vi "固定站流程平行样自动启动.vi"(11 "参数":T1) -> ()   [LabVIEW 2016, in "质控单元.lvlib"]
panel:
  out "枚举":enum16{"初始化", "采配水启动", "等待", "配水", "排水", "结束"}(ring)
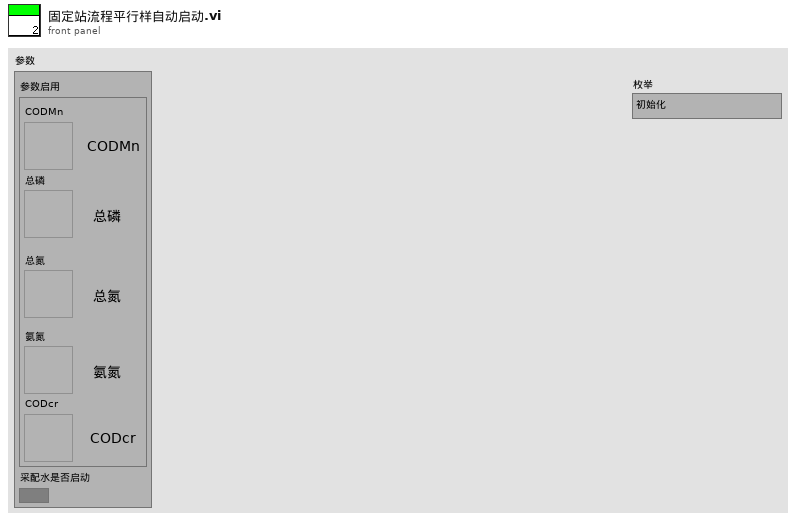
[diagram p1: front panel]
types:
  T1 = cluster{"参数启用":cluster{"CODMn":bool, "总磷":bool, "总氮":bool, "氨氮":bool, "CODcr":bool}, "采配水是否启动":bool}
  T2 = cluster{"命令":string, cluster{"starting address":u16, "holding register value":u16}}
  T3 = typedef "质控单元.lvlib/平行样测试流程.ctl" = enum16{"待机", "第一次水样测试启动", "第一次水样测试中", "第二次水样测试启动", "第二次水样测试中", "存储平行样测试数据", "结束"}
  T4 = cluster{"站号":u16, "量程切换":enum32{"H", "L", "AUTO"}, "控制命令":enum16{"启动测量", "标样核查", "零点核查", "跨度核查", "空白测试", "平行样测试", "加标回收", "空白校准", "标样校准", "初始化（清洗）", "停止测试", "仪器重启", "校时", "模式设置", "测量间隔设置"}, "模式设置":enum16{"待机", "连续模式", "周期模式", "定点模式", "受控模式", "手动模式"}, "测量间隔":u16}
  T5 = cluster{"时间标识":timestamp, "设备":string, "日志信息":string}
  T6 = enum16{"空闲", "水样测试", "标样核查", "零点核查", "跨度核查", "空白测试", "平行样测试", "加标回收", "空白校准", "标样校准", "初始化（清洗）"}
  T7 = cluster{"测量模式":enum16{"水样测量", "标样核查", "零点核查", "跨度核查", "空白测试", "加标回收", "平行样", "校零", "校标"}}
  T8 = cluster{"时间标识":timestamp, "设备":string, "日志信息":string, "流程参数":string}
  T9 = cluster{"R0":i16, "R1":i16, "R2":i16, "R3":i16, "R4":i16, "R5":i16, "R6":i16, "R7":i16, "R8":i16, "R9":i16, "R10":i16, "R11":i16, "R12":i16, "R13":i16, "R14":i16, "R15":i16, "R16":i16, "R17":i16, "R18":i16, "R19":i16, "R20":i16, "R21":i16, "R22":i16, "R23":i16, "R24":i16, "R25":i16, "R26":i16, "R27":i16, "R28":i16, "R29":i16, "R30":i16, "R31":i16, "R32":i16, "R33":i16, "R34":i16, "R35":i16, "R36":i16, "R37":i16, "R38":i16, "R39":i16, "R40":i16, "R41":i16, "R42":i16, "R43":i16, "R44":i16, "R45":i16, "R46":i16, "R47":i16, "R48":i16, "R49":i16, "R50":i16, "R51":i16, "R52":i16, "R53":i16, "R54":i16, "R55":i16, "R56":i16}
  T10 = cluster{"时间标识":timestamp, "参数":string, "数据类型":string, "第一次水样浓度值":sgl, "第二次水样测试时间":timestamp, "第二次水样浓度值":sgl}
  T11 = cluster{"系统时间":timestamp, "工作状态":enum16{"空闲", "水样测试", "标样核查", "零点核查", "跨度核查", "空白测试", "平行样测试", "加标回收", "空白校准", "标样校准", "初始化（清洗）"}, "测量模式":enum16{"待机", "连续模式", "周期模式", "定点模式", "受控模式", "手动模式"}, "告警代码":enum16{"无告警", "缺试剂告警", "缺水样告警", "缺蒸馏水告警", "缺标液告警", "仪表漏液告警", "标定异常告警", "超量程告警", "加热异常", "低试剂预警", "超上限告警", "超下限告警", "仪表内部其他异常", "滴定异常告警", "电极异常告警", "量程切换告警", "参数设置告警", "PH电极电位异常", "电导率电极异常", "浊度光度异常", "溶解氧电极异常", "溶解氧光强异常", "温度异常告警", "PH异常告警", "溶解氧异常告警", "电导率异常告警", "浊度异常告警", "叶绿素异常告警", "藻密度异常告警", "蓝绿藻异常告警", "ORP异常告警", "氨氮异常告警", "清洁刷异常告警", "SD卡异常告警", "蓝牙异常告警", "Wifi异常告警", "流程异常告警"}, "故障代码":enum16{"无故障", "电机故障", "温度故障", "通讯故障", "滴定故障"}, "日志代码":u16, "软件版本":u16, "F0":sgl, "F1":sgl, "F2":sgl, "F3":sgl, "T":sgl, "H":sgl, "id":u16, "flowid":u16, "量程":u16, "总磷控温温度1":sgl, "营养盐控温温度2":sgl, "ADC":sgl}
  T12 = cluster{"因子编码":u32, "单位":u16, "标样参考值":sgl, "水样数据时间":timestamp, "水样实测值":sgl, "水样数据标识":string, "标样数据时间":timestamp, "标样实测值":sgl, "标样数据标识":string, "空白数据时间":timestamp, "空白实测值":sgl, "空白数据标识":string, "零点核查数据时间":timestamp, "零点核查实测值":sgl, "零点核查数据标识":string, "跨度核查数据时间":timestamp, "跨度核查实测值":sgl, "跨度核查数据标识":string, "加标回收数据时间":timestamp, "加标回收实测值":sgl, "加标回收数据标识":string, "平行样数据时间":timestamp, "平行样实测值":sgl, "平行样数据标识":string}
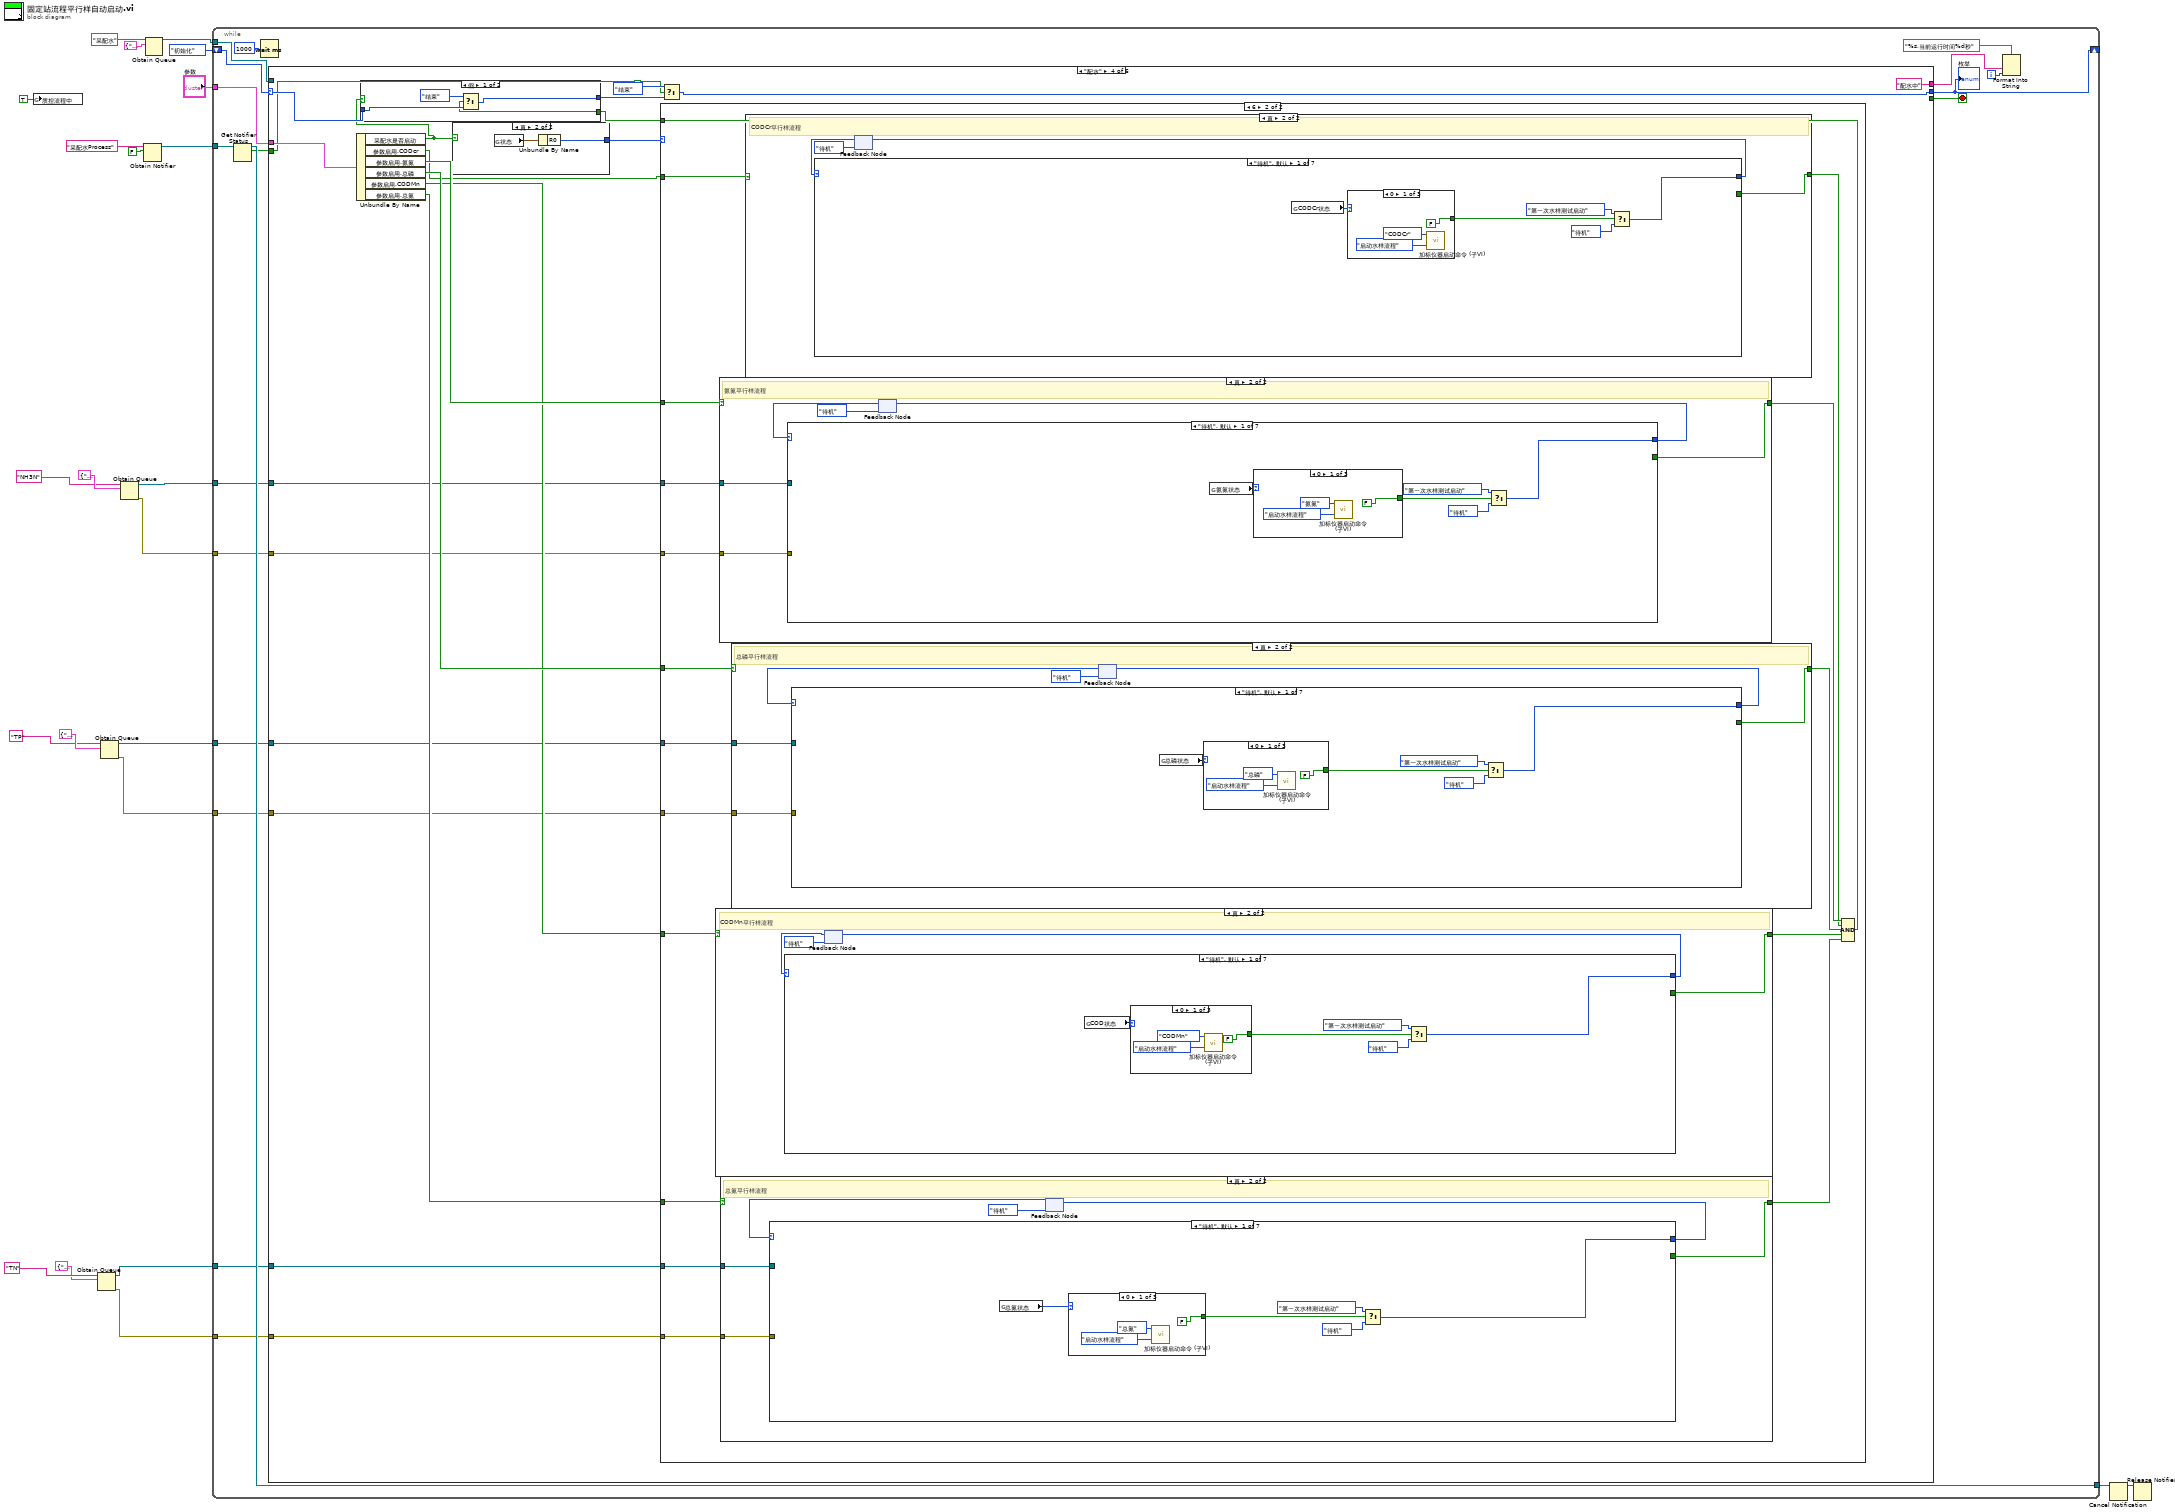
[diagram p0: block diagram]
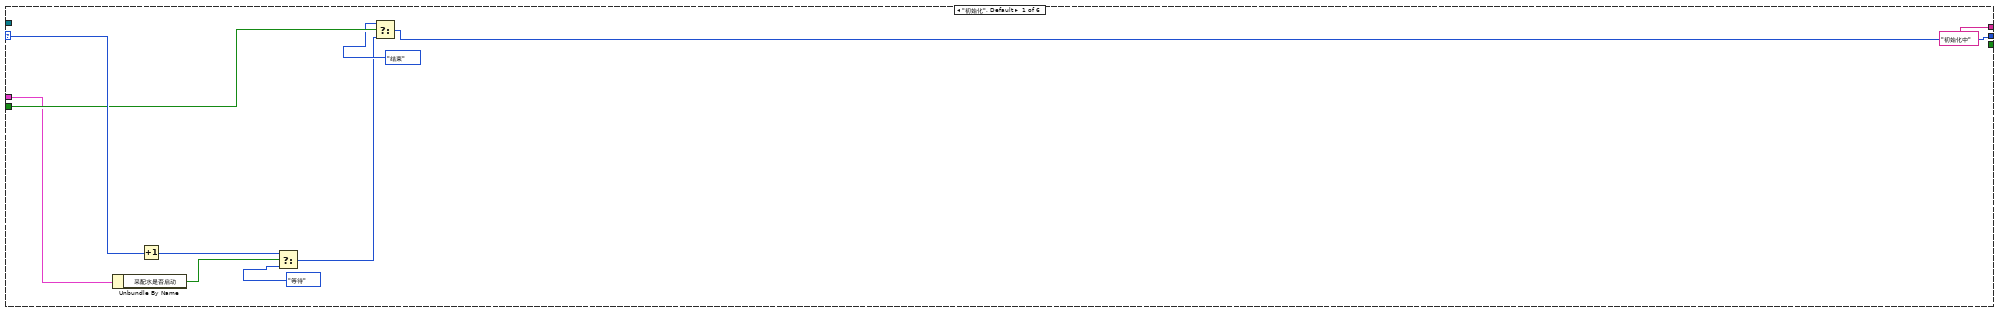
[diagram p2: hidden frame]
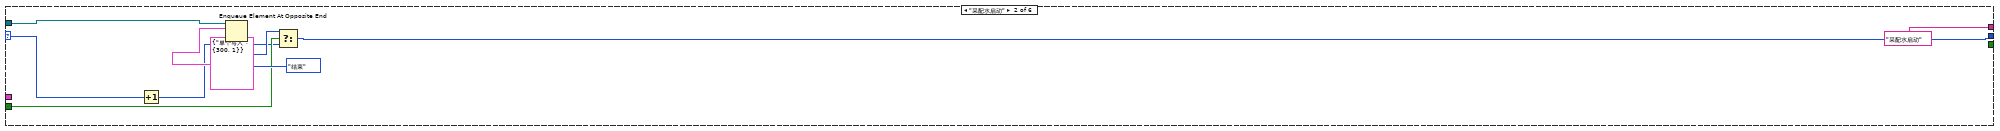
[diagram p3: hidden frame]
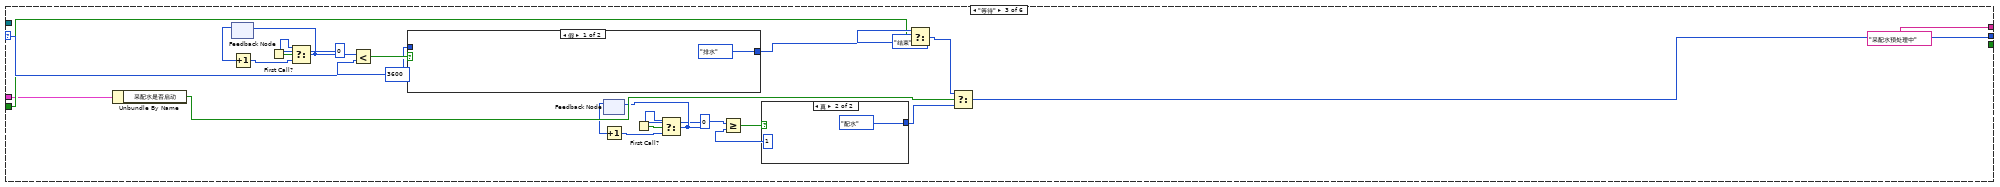
[diagram p4: hidden frame]
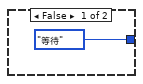
[diagram p5: hidden frame]
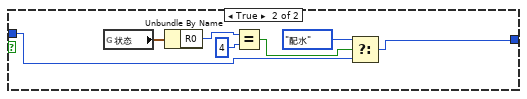
[diagram p6: hidden frame]
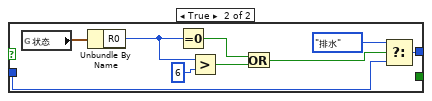
[diagram p7: hidden frame]
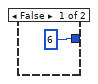
[diagram p8: hidden frame]
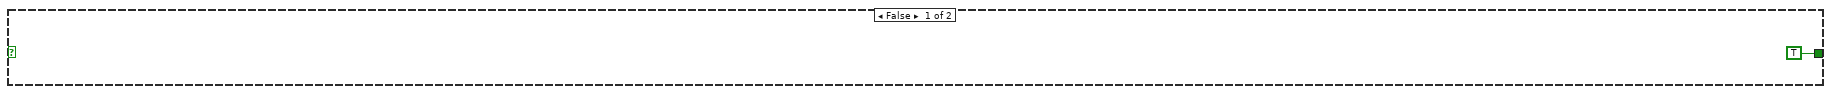
[diagram p10: hidden frame]
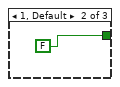
[diagram p11: hidden frame]
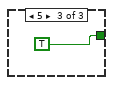
[diagram p12: hidden frame]
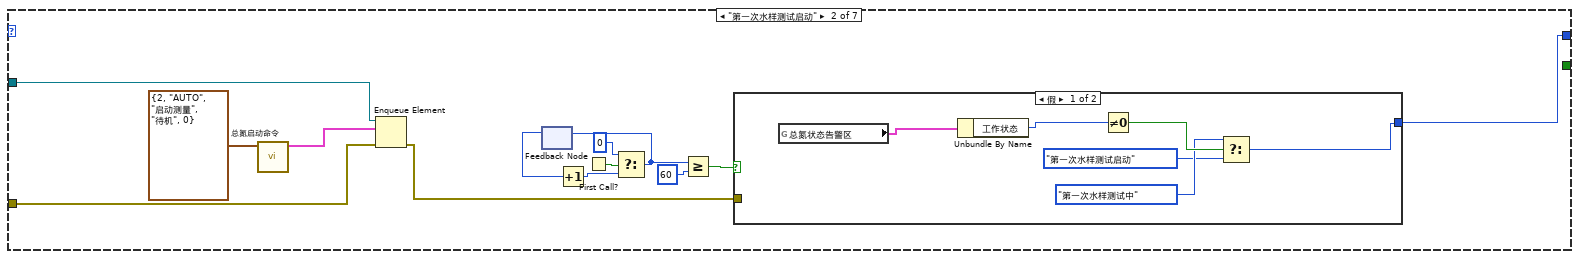
[diagram p13: hidden frame]
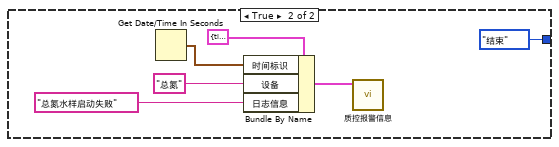
[diagram p14: hidden frame]
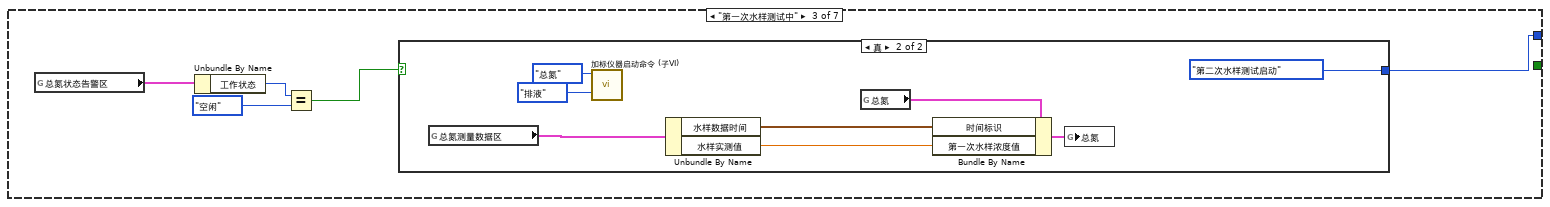
[diagram p15: hidden frame]
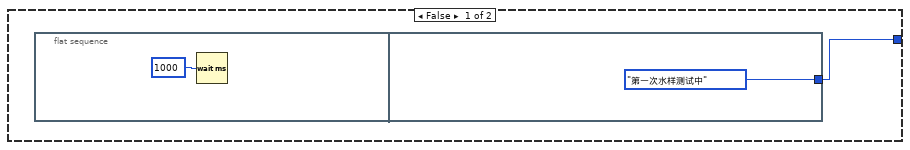
[diagram p16: hidden frame]
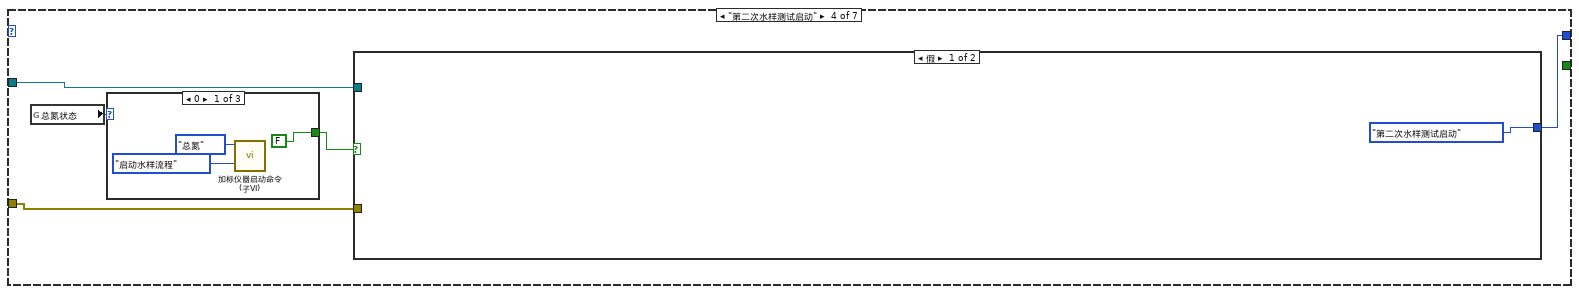
[diagram p17: hidden frame]
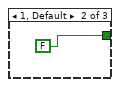
[diagram p18: hidden frame]
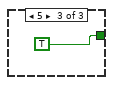
[diagram p19: hidden frame]
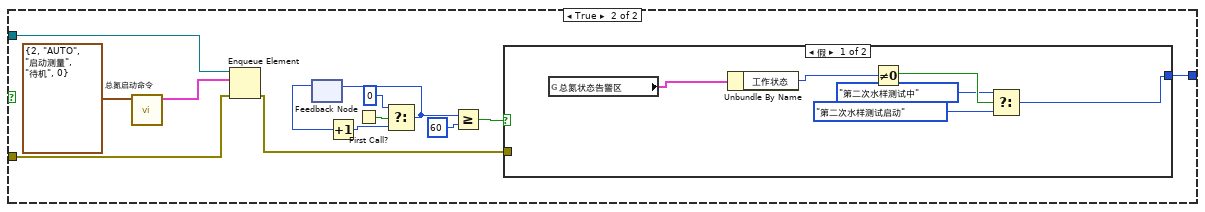
[diagram p20: hidden frame]
diagram:
  n1 = global write "质控测完标志全局 1.vi" "质控流程中"(TRUE ("质控流程中")) -> ()
  n2 = Obtain Queue(name (unnamed)="TN" ("名称（未命名）"), element data type=cluster{"命令":string, "data":variant} {"命令"="", "data"=variant}) -> (queue out=w3:refnum<queue>, error out=w2:errorcluster)  [unwired: 3 in, 1 out]
  n3 = Obtain Queue(name (unnamed)="TP" ("名称（未命名）"), element data type=cluster{"命令":string, "data":variant} {"命令"="", "data"=variant}) -> (queue out=w5:refnum<queue>, error out=w4:errorcluster)  [unwired: 3 in, 1 out]
  n4 = Obtain Queue(name (unnamed)="NH3N" ("名称（未命名）"), element data type=cluster{"命令":string, "data":variant} {"命令"="", "data"=variant}) -> (queue out=w7:refnum<queue>, error out=w6:errorcluster)  [unwired: 3 in, 1 out]
  n5 = Obtain Notifier(name (unnamed)="采配水Process" ("名称（未命名）"), notification data type=FALSE) -> (notifier out=w16:refnum<notifier>)  [unwired: 2 in, 2 out]
  n6 = Obtain Queue(name (unnamed)="采配水" ("名称（未命名）"), element data type=cluster{"命令":string, "数据":variant} {"命令"="", "数据"=variant}) -> (queue out=w21:refnum<queue>)  [unwired: 3 in, 2 out]
  n7 = while {
    tunnel: w21 -> [w41]
    shift-right: [w39] -> _
    shift-left: enum16{"初始化", "采配水启动", "等待", "配水", "排水", "结束"}."初始化" ("枚举") -> [w40]
    tunnel: "参数" -> [w37]
    tunnel: w16 -> [w36]
    tunnel: [w35] -> w15
    tunnel: w7 -> [w30]
    tunnel: w6 -> [w29]
    tunnel: w5 -> [w28]
    tunnel: w4 -> [w27]
    tunnel: w3 -> [w26]
    tunnel: w2 -> [w25]
    i -> [w32]
    stop <- w24 stop-if-true
    n8 = Get Notifier Status(notifier=w36) -> (notifier out=w35:refnum<notifier>, current notification=w31:bool)  [unwired: 1 in, 3 out]
    n9 = Wait (ms)(milliseconds to wait=u32 1000 ("等待时间（毫秒）")) -> ()  [unwired: 1 out]
    n10 = case shown="\"配水\"" w40 {
      selector: w40 -> [w51 w57 w81 w114 w707 w714]
      tunnel: w41 -> [_ w58 _ _ w708 _]
      tunnel: [w48 w52 w60 w111 w702 w713] -> w39
      tunnel: [_ _ _ _ _ TRUE] -> w24
      tunnel: w37 -> [w46 _ w71 w107 _ _]
      tunnel: ["初始化中" ("输入 1") "采配水启动" ("输入 1") "采配水预处理中" ("输入 1") "配水中" ("输入 1") "排水中" ("输入 1") "结束" ("输入 1")] -> w33
      tunnel: w31 -> [w49 w54 w73 w95 w704 _]
      tunnel: w30 -> [_ _ _ w102 _ _]
      tunnel: w29 -> [_ _ _ w101 _ _]
      tunnel: w28 -> [_ _ _ w100 _ _]
      tunnel: w27 -> [_ _ _ w99 _ _]
      tunnel: w26 -> [_ _ _ w98 _ _]
      tunnel: w25 -> [_ _ _ w97 _ _]
      frame "初始化", Default {
        n11 = Unbundle By Name(w46) -> ("采配水是否启动"=w45:bool)
        n12 = Increment(x=w51) -> (x+1=w44:enum16{"初始化", "采配水启动", "等待", "配水", "排水", "结束"})
        n13 = Select(t=w44, s=w45, f=enum16{"初始化", "采配水启动", "等待", "配水", "排水", "结束"}."等待") -> (s? t:f=w43:enum16{"初始化", "采配水启动", "等待", "配水", "排水", "结束"})
        n14 = Select(t=enum16{"初始化", "采配水启动", "等待", "配水", "排水", "结束"}."结束", s=w49, f=w43) -> (s? t:f=w48:enum16{"初始化", "采配水启动", "等待", "配水", "排水", "结束"})
      }
      frame "采配水启动" {
        n15 = Increment(x=w57) -> (x+1=w53:enum16{"初始化", "采配水启动", "等待", "配水", "排水", "结束"})
        n16 = Enqueue Element At Opposite End(queue=w58, element=T2 {"命令"="单个写入", {"starting address"=300, "holding register value"=1}} ("元素")) -> ()  [unwired: 2 in, 3 out]
        n17 = Select(t=enum16{"初始化", "采配水启动", "等待", "配水", "排水", "结束"}."结束", s=w54, f=w53) -> (s? t:f=w52:enum16{"初始化", "采配水启动", "等待", "配水", "排水", "结束"})
      }
      frame "等待" {
        n18 = Unbundle By Name(w71) -> ("采配水是否启动"=w70:bool)
        n19 = feedback #1() -> (w78:i32)  [unwired: 1 in]
        n20 = Increment(x=w78) -> (x+1=w77:i32)
        n21 = First Call?() -> (First Call?: T/F=w79:bool)
        n22 = Select(t=0, s=w79, f=w77) -> (s? t:f=w76:i32)
        n23 = feedback-in #1(w76) -> ()
        n24 = Less?(x=w76, y=3600) -> (x < y?=w82:bool)
        n25 = case shown="假" w82 {
          tunnel: w81 -> [_ w88]
          tunnel: [enum16{"初始化", "采配水启动", "等待", "配水", "排水", "结束"}."排水" ("枚举") w87] -> w72
          frame False {
          }
          frame True {
            n26 = global read "与采配水交互全局.vi" "状态"() -> (w93:T9)
            n27 = Unbundle By Name(w93) -> ("R0"=w92:i16)
            n28 = Equal?(x=w92, y=i16 4) -> (x = y?=w90:bool)
            n29 = Select(t=enum16{"初始化", "采配水启动", "等待", "配水", "排水", "结束"}."配水" ("枚举"), s=w90, f=w88) -> (s? t:f=w87:enum16{"初始化", "采配水启动", "等待", "配水", "排水", "结束"})
          }
        }
        n30 = feedback #2() -> (w66:i32)  [unwired: 1 in]
        n31 = Increment(x=w66) -> (x+1=w67:i32)
        n32 = First Call?() -> (First Call?: T/F=w65:bool)
        n33 = Select(t=0, s=w65, f=w67) -> (s? t:f=w68:i32)
        n34 = feedback-in #2(w68) -> ()
        n35 = Greater Or Equal?(x=w68, y=1) -> (x >= y?=w62:bool)
        n36 = case shown="真" w62 {
          tunnel: [enum16{"初始化", "采配水启动", "等待", "配水", "排水", "结束"}."等待" ("t") enum16{"初始化", "采配水启动", "等待", "配水", "排水", "结束"}."配水" ("t")] -> w61
          frame False {
          }
          frame True {
          }
        }
        n37 = Select(t=enum16{"初始化", "采配水启动", "等待", "配水", "排水", "结束"}."结束", s=w73, f=w72) -> (s? t:f=w69:enum16{"初始化", "采配水启动", "等待", "配水", "排水", "结束"})
        n38 = Select(t=w69, s=w70, f=w61) -> (s? t:f=w60:enum16{"初始化", "采配水启动", "等待", "配水", "排水", "结束"})
      }
      frame "配水" {
        n39 = Unbundle By Name(w107) -> ("采配水是否启动"=w96:bool, "参数启用.CODcr"=w106:bool, "参数启用.氨氮"=w110:bool, "参数启用.总磷"=w109:bool, "参数启用.CODMn"=w108:bool, "参数启用.总氮"=w105:bool)
        n40 = case shown="真" w96 {
          tunnel: [i16 6 ("R0") w129] -> w104
          frame False {
          }
          frame True {
            n41 = global read "与采配水交互全局.vi" "状态"() -> (w130:T9)
            n42 = Unbundle By Name(w130) -> ("R0"=w129:i16)
          }
        }
        n43 = case shown="6" w104 {
          tunnel: w110 -> [_ w147]
          tunnel: w109 -> [_ w146]
          tunnel: w108 -> [_ w143]
          tunnel: w106 -> [_ w142]
          tunnel: w105 -> [_ w139]
          tunnel: w102 -> [_ w137]
          tunnel: w101 -> [_ w136]
          tunnel: w100 -> [_ w135]
          tunnel: w99 -> [_ w134]
          tunnel: w98 -> [_ w133]
          tunnel: w97 -> [_ w132]
          tunnel: [_ w131] -> w94
          frame 0, Default {
          }
          frame 6 {
            n44 = case shown="真" w143 {
              tunnel: [TRUE w264] -> w140
              frame False {
              }
              frame True {
                # "CODMn平行样流程"
                n45 = feedback #3(平行样测试流程."待机") -> (w266:T3)
                n46 = case shown="\"待机\", 默认" w266 {
                  tunnel: [w267 w286 w300 w313 w343 平行样测试流程."结束" 平行样测试流程."结束"] -> w265
                  tunnel: [_ _ _ _ _ _ TRUE] -> w264
                  frame "待机", Default {
                    n47 = global read "加标回收状态全局变量.vi" "COD状态"() -> (w271:u16)
                    n48 = case shown="0" w271 {
                      tunnel: [FALSE ("s") FALSE ("s") TRUE ("s")] -> w270
                      frame 0 {
                        n49 = call "加标仪器启动命令 (子VI).vi"("启动命令"=enum16{"启动水样流程", "启动加标流程", "排液", "停止"}."启动水样流程", "仪器"=enum16{"", "氨氮", "总磷", "总氮", "CODMn", "CODCr"}."CODMn") -> ()  [unwired: 9 in, 1 out]
                      }
                      frame 1, Default {
                      }
                      frame 5 {
                      }
                    }
                    n50 = Select(t=平行样测试流程."第一次水样测试启动", s=w270, f=平行样测试流程."待机") -> (s? t:f=w267:T3)
                  }
                  frame "第一次水样测试启动" {
                    n51 = feedback #4() -> (w282:i32)  [unwired: 1 in]
                    n52 = Increment(x=w282) -> (x+1=w283:i32)
                    n53 = call "CODMn启动命令 (子VI).vi"("启动测量模式"=T7 {"测量模式"=enum."水样测量"}) -> ("错误输出"=w277:errorcluster)  [unwired: 10 in]
                    n54 = First Call?() -> (First Call?: T/F=w281:bool)
                    n55 = Select(t=0, s=w281, f=w283) -> (s? t:f=w284:i32)
                    n56 = feedback-in #4(w284) -> ()
                    n57 = Greater Or Equal?(x=w284, y=60) -> (x >= y?=w279:bool)
                    n58 = case shown="假" w279 {
                      tunnel: [w290 平行样测试流程."结束"] -> w286
                      tunnel: w277 -> [_ _]
                      frame False {
                        n59 = global read "与CODMn交互全局.vi" "多列列表框"() -> (w289:i32)
                        n60 = Not Equal To 0?(x=w289) -> (x != 0?=w291:bool)
                        n61 = Select(t=平行样测试流程."第一次水样测试中", s=w291, f=平行样测试流程."第一次水样测试启动") -> (s? t:f=w290:T3)
                      }
                      frame True {
                        n62 = Get Date/Time In Seconds() -> (seconds since 1Jan1904=w294:timestamp)
                        n63 = Bundle By Name(cluster=T5 {"时间标识"=timestamp(0 s since 1904-01-01), "设备"="", "日志信息"=""} ("data in"), "时间标识"=w294, "设备"="CODMn", "日志信息"="CODMn启动失败") -> (w292:T5)
                        n64 = call "质控报警信息.vi"("data in"=w292) -> ()  [unwired: 10 in, 1 out]
                      }
                    }
                  }
                  frame "第一次水样测试中" {
                    n65 = global read "与CODMn交互全局.vi" "多列列表框"() -> (w299:i32)
                    n66 = Equal To 0?(x=w299) -> (x = 0?=w298:bool)
                    n67 = case shown="真" w298 {
                      tunnel: [w301 平行样测试流程."第二次水样测试启动"] -> w300
                      frame False {
                        n68 = flat-sequence {
                          tunnel: [平行样测试流程."第一次水样测试中"] -> w301
                          frame #0 {
                            n69 = Wait (ms)(milliseconds to wait=u32 1000 ("等待时间（毫秒）")) -> ()  [unwired: 1 out]
                          }
                          frame #1 {
                          }
                        }
                      }
                      frame True {
                        n70 = global read "与CODMn交互全局.vi" "COD浓度（mg/L)"() -> (w306:dbl)
                        n71 = global read "与CODMn交互全局.vi" "水样启动时间"() -> (w307:timestamp)
                        n72 = global read "平行样测试全局变量.vi" "CODMn"() -> (w309:T10)
                        n73 = Bundle By Name(cluster=w309, "时间标识"=w307, "第一次水样浓度值"=w306) -> (w308:T10)
                        n74 = global write "平行样测试全局变量.vi" "CODMn"(w308) -> ()
                        n75 = call "加标仪器启动命令 (子VI).vi"("启动命令"=enum16{"启动水样流程", "启动加标流程", "排液", "停止"}."排液", "仪器"=enum16{"", "氨氮", "总磷", "总氮", "CODMn", "CODCr"}."CODMn") -> ()  [unwired: 9 in, 1 out]
                      }
                    }
                  }
                  frame "第二次水样测试启动" {
                    n76 = global read "加标回收状态全局变量.vi" "COD状态"() -> (w312:u16)
                    n77 = case shown="0" w312 {
                      tunnel: [FALSE ("s") FALSE ("s") TRUE ("s")] -> w311
                      frame 0 {
                        n78 = call "加标仪器启动命令 (子VI).vi"("启动命令"=enum16{"启动水样流程", "启动加标流程", "排液", "停止"}."启动水样流程", "仪器"=enum16{"", "氨氮", "总磷", "总氮", "CODMn", "CODCr"}."CODMn") -> ()  [unwired: 9 in, 1 out]
                      }
                      frame 1, Default {
                      }
                      frame 5 {
                      }
                    }
                    n79 = case shown="真" w311 {
                      tunnel: [平行样测试流程."第二次水样测试启动" w324] -> w313
                      frame False {
                      }
                      frame True {
                        n80 = feedback #5() -> (w320:i32)  [unwired: 1 in]
                        n81 = Increment(x=w320) -> (x+1=w321:i32)
                        n82 = First Call?() -> (First Call?: T/F=w319:bool)
                        n83 = call "CODMn启动命令 (子VI).vi"("启动测量模式"=T7 {"测量模式"=enum."水样测量"}) -> ("错误输出"=w315:errorcluster)  [unwired: 10 in]
                        n84 = Select(t=0, s=w319, f=w321) -> (s? t:f=w322:i32)
                        n85 = feedback-in #5(w322) -> ()
                        n86 = Greater Or Equal?(x=w322, y=60) -> (x >= y?=w317:bool)
                        n87 = case shown="真" w317 {
                          tunnel: [w328 平行样测试流程."结束"] -> w324
                          tunnel: w315 -> [_ _]
                          frame False {
                            n88 = global read "与CODMn交互全局.vi" "多列列表框"() -> (w327:i32)
                            n89 = Not Equal To 0?(x=w327) -> (x != 0?=w329:bool)
                            n90 = Select(t=平行样测试流程."第二次水样测试中", s=w329, f=平行样测试流程."第二次水样测试启动") -> (s? t:f=w328:T3)
                          }
                          frame True {
                            n91 = Get Date/Time In Seconds() -> (seconds since 1Jan1904=w332:timestamp)
                            n92 = Bundle By Name(cluster=T5 {"时间标识"=timestamp(0 s since 1904-01-01), "设备"="", "日志信息"=""} ("data in"), "时间标识"=w332, "设备"="CODMn", "日志信息"="CODMn启动失败") -> (w330:T5)
                            n93 = call "质控报警信息.vi"("data in"=w330) -> ()  [unwired: 10 in, 1 out]
                          }
                        }
                      }
                    }
                  }
                  frame "第二次水样测试中" {
                    n94 = global read "与CODMn交互全局.vi" "多列列表框"() -> (w342:i32)
                    n95 = Equal To 0?(x=w342) -> (x = 0?=w341:bool)
                    n96 = case shown="真" w341 {
                      tunnel: [w344 平行样测试流程."存储平行样测试数据"] -> w343
                      frame False {
                        n97 = flat-sequence {
                          tunnel: [平行样测试流程."第二次水样测试中"] -> w344
                          frame #0 {
                            n98 = Wait (ms)(milliseconds to wait=u32 1000 ("等待时间（毫秒）")) -> ()  [unwired: 1 out]
                          }
                          frame #1 {
                          }
                        }
                      }
                      frame True {
                        n99 = global read "与CODMn交互全局.vi" "COD浓度（mg/L)"() -> (w349:dbl)
                        n100 = global read "与CODMn交互全局.vi" "水样启动时间"() -> (w350:timestamp)
                        n101 = global read "平行样测试全局变量.vi" "CODMn"() -> (w352:T10)
                        n102 = Bundle By Name(cluster=w352, "时间标识"=w350, "第一次水样浓度值"=w349) -> (w351:T10)
                        n103 = global write "平行样测试全局变量.vi" "CODMn"(w351) -> ()
                        n104 = call "加标仪器启动命令 (子VI).vi"("启动命令"=enum16{"启动水样流程", "启动加标流程", "排液", "停止"}."排液", "仪器"=enum16{"", "氨氮", "总磷", "总氮", "CODMn", "CODCr"}."CODMn") -> ()  [unwired: 9 in, 1 out]
                      }
                    }
                  }
                  frame "存储平行样测试数据" {
                    n105 = global read "平行样测试全局变量.vi" "CODMn"() -> (w354:T10)
                    n106 = call "平行样测试数据写入.vi"("data"=w354) -> ()  [unwired: 10 in, 1 out]
                  }
                  frame "结束" {
                  }
                }
                n107 = feedback-in #3(w265) -> ()
              }
            }
            n108 = case shown="真" w147 {
              tunnel: [TRUE w592] -> w145
              tunnel: w137 -> [_ w591]
              tunnel: w136 -> [_ w590]
              frame False {
              }
              frame True {
                # "氨氮平行样流程"
                n109 = feedback #6(平行样测试流程."待机") -> (w594:T3)
                n110 = case shown="\"待机\", 默认" w594 {
                  tunnel: [w596 w606 w635 w651 w686 平行样测试流程."结束" 平行样测试流程."结束"] -> w593
                  tunnel: [_ _ _ _ _ _ TRUE] -> w592
                  tunnel: w591 -> [_ w616 _ w650 _ _ _]
                  tunnel: w590 -> [_ w615 _ w649 _ _ _]
                  frame "待机", Default {
                    n111 = global read "加标回收状态全局变量.vi" "氨氮状态"() -> (w600:u16)
                    n112 = case shown="0" w600 {
                      tunnel: [FALSE ("s") FALSE ("s") TRUE ("s")] -> w599
                      frame 0 {
                        n113 = call "加标仪器启动命令 (子VI).vi"("启动命令"=enum16{"启动水样流程", "启动加标流程", "排液", "停止"}."启动水样流程", "仪器"=enum16{"", "氨氮", "总磷", "总氮", "CODMn", "CODCr"}."氨氮") -> ()  [unwired: 9 in, 1 out]
                      }
                      frame 1, Default {
                      }
                      frame 5 {
                      }
                    }
                    n114 = Select(t=平行样测试流程."第一次水样测试启动", s=w599, f=平行样测试流程."待机") -> (s? t:f=w596:T3)
                  }
                  frame "第一次水样测试启动" {
                    n115 = call "氨氮启动命令.vi"("参数"=T4 {"站号"=3, "量程切换"=enum."AUTO", "控制命令"=enum."启动测量", "模式设置"=enum."受控模式", "测量间隔"=0}) -> ("启动命令"=w618:cluster{"命令":string, "data":variant})  [unwired: 10 in]
                    n116 = Enqueue Element(queue=w616, element=w618, error in (no error)=w615) -> (error out=w607:errorcluster)  [unwired: 1 in, 2 out]
                    n117 = feedback #7() -> (w611:i32)  [unwired: 1 in]
                    n118 = Increment(x=w611) -> (x+1=w612:i32)
                    n119 = First Call?() -> (First Call?: T/F=w610:bool)
                    n120 = Select(t=0, s=w610, f=w612) -> (s? t:f=w613:i32)
                    n121 = feedback-in #7(w613) -> ()
                    n122 = Greater Or Equal?(x=w613, y=60) -> (x >= y?=w608:bool)
                    n123 = case shown="假" w608 {
                      tunnel: [w623 平行样测试流程."结束"] -> w606
                      tunnel: w607 -> [_ _]
                      frame False {
                        n124 = global read "与氨氮交互全局.vi" "氨氮状态告警区"() -> (w619:T11)
                        n125 = Unbundle By Name(w619) -> ("工作状态"=w620:T6)
                        n126 = Not Equal To 0?(x=w620) -> (x != 0?=w624:bool)
                        n127 = Select(t=平行样测试流程."第一次水样测试中", s=w624, f=平行样测试流程."第一次水样测试启动") -> (s? t:f=w623:T3)
                      }
                      frame True {
                        n128 = Get Date/Time In Seconds() -> (seconds since 1Jan1904=w627:timestamp)
                        n129 = Bundle By Name(cluster=T5 {"时间标识"=timestamp(0 s since 1904-01-01), "设备"="", "日志信息"=""} ("data in"), "时间标识"=w627, "设备"="氨氮", "日志信息"="氨氮水样启动失败") -> (w625:T5)
                        n130 = call "质控报警信息.vi"("data in"=w625) -> ()  [unwired: 10 in, 1 out]
                      }
                    }
                  }
                  frame "第一次水样测试中" {
                    n131 = global read "与氨氮交互全局.vi" "氨氮状态告警区"() -> (w634:T11)
                    n132 = Unbundle By Name(w634) -> ("工作状态"=w632:T6)
                    n133 = Equal?(x=w632, y=T6."空闲" ("工作状态")) -> (x = y?=w631:bool)
                    n134 = case shown="真" w631 {
                      tunnel: [w636 平行样测试流程."第二次水样测试启动"] -> w635
                      frame False {
                        n135 = flat-sequence {
                          tunnel: [平行样测试流程."第一次水样测试中"] -> w636
                          frame #0 {
                            n136 = Wait (ms)(milliseconds to wait=u32 1000 ("等待时间（毫秒）")) -> ()  [unwired: 1 out]
                          }
                          frame #1 {
                          }
                        }
                      }
                      frame True {
                        n137 = call "加标仪器启动命令 (子VI).vi"("启动命令"=enum16{"启动水样流程", "启动加标流程", "排液", "停止"}."排液", "仪器"=enum16{"", "氨氮", "总磷", "总氮", "CODMn", "CODCr"}."氨氮") -> ()  [unwired: 9 in, 1 out]
                        n138 = global read "与氨氮交互全局.vi" "氨氮测量数据区"() -> (w643:T12)
                        n139 = Unbundle By Name(w643) -> ("水样数据时间"=w642:timestamp, "水样实测值"=w641:sgl)
                        n140 = global read "平行样测试全局变量.vi" "氨氮"() -> (w645:T10)
                        n141 = Bundle By Name(cluster=w645, "时间标识"=w642, "第一次水样浓度值"=w641) -> (w644:T10)
                        n142 = global write "平行样测试全局变量.vi" "氨氮"(w644) -> ()
                      }
                    }
                  }
                  frame "第二次水样测试启动" {
                    n143 = global read "加标回收状态全局变量.vi" "氨氮状态"() -> (w648:u16)
                    n144 = case shown="0" w648 {
                      tunnel: [FALSE ("s") FALSE ("s") TRUE ("s")] -> w647
                      frame 0 {
                        n145 = call "加标仪器启动命令 (子VI).vi"("启动命令"=enum16{"启动水样流程", "启动加标流程", "排液", "停止"}."启动水样流程", "仪器"=enum16{"", "氨氮", "总磷", "总氮", "CODMn", "CODCr"}."氨氮") -> ()  [unwired: 9 in, 1 out]
                      }
                      frame 1, Default {
                      }
                      frame 5 {
                      }
                    }
                    n146 = case shown="真" w647 {
                      tunnel: [平行样测试流程."第二次水样测试启动" w662] -> w651
                      tunnel: w650 -> [_ w659]
                      tunnel: w649 -> [_ w658]
                      frame False {
                      }
                      frame True {
                        n147 = call "氨氮启动命令.vi"("参数"=T4 {"站号"=3, "量程切换"=enum."AUTO", "控制命令"=enum."启动测量", "模式设置"=enum."受控模式", "测量间隔"=0}) -> ("启动命令"=w661:cluster{"命令":string, "data":variant})  [unwired: 10 in]
                        n148 = Enqueue Element(queue=w659, element=w661, error in (no error)=w658) -> ()  [unwired: 1 in, 3 out]
                        n149 = feedback #8() -> (w666:i32)  [unwired: 1 in]
                        n150 = Increment(x=w666) -> (x+1=w667:i32)
                        n151 = First Call?() -> (First Call?: T/F=w665:bool)
                        n152 = Select(t=0, s=w665, f=w667) -> (s? t:f=w668:i32)
                        n153 = feedback-in #8(w668) -> ()
                        n154 = Greater Or Equal?(x=w668, y=60) -> (x >= y?=w663:bool)
                        n155 = case shown="假" w663 {
                          tunnel: [w672 平行样测试流程."结束"] -> w662
                          frame False {
                            n156 = global read "与氨氮交互全局.vi" "氨氮状态告警区"() -> (w675:T11)
                            n157 = Unbundle By Name(w675) -> ("工作状态"=w671:T6)
                            n158 = Not Equal To 0?(x=w671) -> (x != 0?=w670:bool)
                            n159 = Select(t=平行样测试流程."第二次水样测试中", s=w670, f=平行样测试流程."第二次水样测试启动") -> (s? t:f=w672:T3)
                          }
                          frame True {
                            n160 = Get Date/Time In Seconds() -> (seconds since 1Jan1904=w678:timestamp)
                            n161 = Bundle By Name(cluster=T5 {"时间标识"=timestamp(0 s since 1904-01-01), "设备"="", "日志信息"=""} ("data in"), "时间标识"=w678, "设备"="氨氮", "日志信息"="氨氮水样启动失败") -> (w677:T5)
                            n162 = call "质控报警信息.vi"("data in"=w677) -> ()  [unwired: 10 in, 1 out]
                          }
                        }
                      }
                    }
                  }
                  frame "第二次水样测试中" {
                    n163 = global read "与氨氮交互全局.vi" "氨氮状态告警区"() -> (w685:T11)
                    n164 = Unbundle By Name(w685) -> ("工作状态"=w683:T6)
                    n165 = Equal?(x=w683, y=T6."空闲" ("工作状态")) -> (x = y?=w682:bool)
                    n166 = case shown="真" w682 {
                      tunnel: [w687 平行样测试流程."存储平行样测试数据"] -> w686
                      frame False {
                        n167 = flat-sequence {
                          tunnel: [平行样测试流程."第二次水样测试中"] -> w687
                          frame #0 {
                            n168 = Wait (ms)(milliseconds to wait=u32 1000 ("等待时间（毫秒）")) -> ()  [unwired: 1 out]
                          }
                          frame #1 {
                          }
                        }
                      }
                      frame True {
                        n169 = call "加标仪器启动命令 (子VI).vi"("启动命令"=enum16{"启动水样流程", "启动加标流程", "排液", "停止"}."排液", "仪器"=enum16{"", "氨氮", "总磷", "总氮", "CODMn", "CODCr"}."氨氮") -> ()  [unwired: 9 in, 1 out]
                        n170 = global read "与氨氮交互全局.vi" "氨氮测量数据区"() -> (w694:T12)
                        n171 = Unbundle By Name(w694) -> ("水样数据时间"=w693:timestamp, "水样实测值"=w692:sgl)
                        n172 = global read "平行样测试全局变量.vi" "氨氮"() -> (w696:T10)
                        n173 = Bundle By Name(cluster=w696, "第二次水样测试时间"=w693, "第二次水样浓度值"=w692) -> (w695:T10)
                        n174 = global write "平行样测试全局变量.vi" "氨氮"(w695) -> ()
                      }
                    }
                  }
                  frame "存储平行样测试数据" {
                    n175 = global read "平行样测试全局变量.vi" "氨氮"() -> (w698:T10)
                    n176 = call "平行样测试数据写入.vi"("data"=w698) -> ()  [unwired: 10 in, 1 out]
                  }
                  frame "结束" {
                  }
                }
                n177 = feedback-in #6(w593) -> ()
              }
            }
            n178 = case shown="真" w139 {
              tunnel: [TRUE w152] -> w138
              tunnel: w133 -> [_ w150]
              tunnel: w132 -> [_ w149]
              frame False {
              }
              frame True {
                # "总氮平行样流程"
                n179 = feedback #9(平行样测试流程."待机") -> (w154:T3)
                n180 = case shown="\"待机\", 默认" w154 {
                  tunnel: [w155 w165 w191 w208 w242 平行样测试流程."结束" 平行样测试流程."结束"] -> w153
                  tunnel: [_ _ _ _ _ _ TRUE] -> w152
                  tunnel: w150 -> [_ w169 _ w210 _ _ _]
                  tunnel: w149 -> [_ w168 _ w209 _ _ _]
                  frame "待机", Default {
                    n181 = global read "加标回收状态全局变量.vi" "总氮状态"() -> (w159:u16)
                    n182 = case shown="0" w159 {
                      tunnel: [FALSE ("s") FALSE ("s") TRUE ("s")] -> w158
                      frame 0 {
                        n183 = call "加标仪器启动命令 (子VI).vi"("启动命令"=enum16{"启动水样流程", "启动加标流程", "排液", "停止"}."启动水样流程", "仪器"=enum16{"", "氨氮", "总磷", "总氮", "CODMn", "CODCr"}."总氮") -> ()  [unwired: 9 in, 1 out]
                      }
                      frame 1, Default {
                      }
                      frame 5 {
                      }
                    }
                    n184 = Select(t=平行样测试流程."第一次水样测试启动", s=w158, f=平行样测试流程."待机") -> (s? t:f=w155:T3)
                  }
                  frame "第一次水样测试启动" {
                    n185 = call "总氮启动命令.vi"("参数"=T4 {"站号"=2, "量程切换"=enum."AUTO", "控制命令"=enum."启动测量", "模式设置"=enum."待机", "测量间隔"=0}) -> ("启动命令"=w167:cluster{"命令":string, "data":variant})  [unwired: 10 in]
                    n186 = Enqueue Element(queue=w169, element=w167, error in (no error)=w168) -> (error out=w170:errorcluster)  [unwired: 1 in, 2 out]
                    n187 = feedback #10() -> (w174:i32)  [unwired: 1 in]
                    n188 = Increment(x=w174) -> (x+1=w173:i32)
                    n189 = First Call?() -> (First Call?: T/F=w175:bool)
                    n190 = Select(t=0, s=w175, f=w173) -> (s? t:f=w172:i32)
                    n191 = feedback-in #10(w172) -> ()
                    n192 = Greater Or Equal?(x=w172, y=60) -> (x >= y?=w177:bool)
                    n193 = case shown="假" w177 {
                      tunnel: [w182 平行样测试流程."结束"] -> w165
                      tunnel: w170 -> [_ _]
                      frame False {
                        n194 = global read "与总氮交互全局.vi" "总氮状态告警区"() -> (w178:T11)
                        n195 = Unbundle By Name(w178) -> ("工作状态"=w179:T6)
                        n196 = Not Equal To 0?(x=w179) -> (x != 0?=w183:bool)
                        n197 = Select(t=平行样测试流程."第一次水样测试中", s=w183, f=平行样测试流程."第一次水样测试启动") -> (s? t:f=w182:T3)
                      }
                      frame True {
                        n198 = Get Date/Time In Seconds() -> (seconds since 1Jan1904=w186:timestamp)
                        n199 = Bundle By Name(cluster=T5 {"时间标识"=timestamp(0 s since 1904-01-01), "设备"="", "日志信息"=""} ("data in"), "时间标识"=w186, "设备"="总氮", "日志信息"="总氮水样启动失败") -> (w184:T5)
                        n200 = call "质控报警信息.vi"("data in"=w184) -> ()  [unwired: 10 in, 1 out]
                      }
                    }
                  }
                  frame "第一次水样测试中" {
                    n201 = global read "与总氮交互全局.vi" "总氮状态告警区"() -> (w190:T11)
                    n202 = Unbundle By Name(w190) -> ("工作状态"=w194:T6)
                    n203 = Equal?(x=w194, y=T6."空闲" ("工作状态")) -> (x = y?=w192:bool)
                    n204 = case shown="真" w192 {
                      tunnel: [w195 平行样测试流程."第二次水样测试启动"] -> w191
                      frame False {
                        n205 = flat-sequence {
                          tunnel: [平行样测试流程."第一次水样测试中"] -> w195
                          frame #0 {
                            n206 = Wait (ms)(milliseconds to wait=u32 1000 ("等待时间（毫秒）")) -> ()  [unwired: 1 out]
                          }
                          frame #1 {
                          }
                        }
                      }
                      frame True {
                        n207 = global read "与总氮交互全局.vi" "总氮测量数据区"() -> (w200:T12)
                        n208 = call "加标仪器启动命令 (子VI).vi"("启动命令"=enum16{"启动水样流程", "启动加标流程", "排液", "停止"}."排液", "仪器"=enum16{"", "氨氮", "总磷", "总氮", "CODMn", "CODCr"}."总氮") -> ()  [unwired: 9 in, 1 out]
                        n209 = Unbundle By Name(w200) -> ("水样数据时间"=w203:timestamp, "水样实测值"=w204:sgl)
                        n210 = global read "平行样测试全局变量.vi" "总氮"() -> (w201:T10)
                        n211 = Bundle By Name(cluster=w201, "时间标识"=w203, "第一次水样浓度值"=w204) -> (w202:T10)
                        n212 = global write "平行样测试全局变量.vi" "总氮"(w202) -> ()
                      }
                    }
                  }
                  frame "第二次水样测试启动" {
                    n213 = global read "加标回收状态全局变量.vi" "总氮状态"() -> (w207:u16)
                    n214 = case shown="0" w207 {
                      tunnel: [FALSE ("s") FALSE ("s") TRUE ("s")] -> w206
                      frame 0 {
                        n215 = call "加标仪器启动命令 (子VI).vi"("启动命令"=enum16{"启动水样流程", "启动加标流程", "排液", "停止"}."启动水样流程", "仪器"=enum16{"", "氨氮", "总磷", "总氮", "CODMn", "CODCr"}."总氮") -> ()  [unwired: 9 in, 1 out]
                      }
                      frame 1, Default {
                      }
                      frame 5 {
                      }
                    }
                    n216 = case shown="假" w206 {
                      tunnel: w210 -> [_ w219]
                      tunnel: w209 -> [_ w218]
                      tunnel: [平行样测试流程."第二次水样测试启动" w217] -> w208
                      frame False {
                      }
                      frame True {
                        n217 = call "总氮启动命令.vi"("参数"=T4 {"站号"=2, "量程切换"=enum."AUTO", "控制命令"=enum."启动测量", "模式设置"=enum."待机", "测量间隔"=0}) -> ("启动命令"=w221:cluster{"命令":string, "data":variant})  [unwired: 10 in]
                        n218 = Enqueue Element(queue=w219, element=w221, error in (no error)=w218) -> (error out=w222:errorcluster)  [unwired: 1 in, 2 out]
                        n219 = feedback #11() -> (w226:i32)  [unwired: 1 in]
                        n220 = Increment(x=w226) -> (x+1=w225:i32)
                        n221 = First Call?() -> (First Call?: T/F=w227:bool)
                        n222 = Select(t=0, s=w227, f=w225) -> (s? t:f=w224:i32)
                        n223 = feedback-in #11(w224) -> ()
                        n224 = Greater Or Equal?(x=w224, y=60) -> (x >= y?=w229:bool)
                        n225 = case shown="假" w229 {
                          tunnel: [w234 平行样测试流程."结束"] -> w217
                          tunnel: w222 -> [_ _]
                          frame False {
                            n226 = global read "与总氮交互全局.vi" "总氮状态告警区"() -> (w230:T11)
                            n227 = Unbundle By Name(w230) -> ("工作状态"=w231:T6)
                            n228 = Not Equal To 0?(x=w231) -> (x != 0?=w235:bool)
                            n229 = Select(t=平行样测试流程."第二次水样测试中", s=w235, f=平行样测试流程."第二次水样测试启动") -> (s? t:f=w234:T3)
                          }
                          frame True {
                            n230 = Get Date/Time In Seconds() -> (seconds since 1Jan1904=w238:timestamp)
                            n231 = Bundle By Name(cluster=T5 {"时间标识"=timestamp(0 s since 1904-01-01), "设备"="", "日志信息"=""} ("data in"), "时间标识"=w238, "设备"="总氮", "日志信息"="总氮水样启动失败") -> (w236:T5)
                            n232 = call "质控报警信息.vi"("data in"=w236) -> ()  [unwired: 10 in, 1 out]
                          }
                        }
                      }
                    }
                  }
                  frame "第二次水样测试中" {
                    n233 = global read "与总氮交互全局.vi" "总氮状态告警区"() -> (w243:T11)
                    n234 = Unbundle By Name(w243) -> ("工作状态"=w246:T6)
                    n235 = Equal?(x=w246, y=T6."空闲" ("工作状态")) -> (x = y?=w244:bool)
                    n236 = case shown="真" w244 {
                      tunnel: [w247 平行样测试流程."存储平行样测试数据"] -> w242
                      frame False {
                        n237 = flat-sequence {
                          tunnel: [平行样测试流程."第二次水样测试中"] -> w247
                          frame #0 {
                            n238 = Wait (ms)(milliseconds to wait=u32 1000 ("等待时间（毫秒）")) -> ()  [unwired: 1 out]
                          }
                          frame #1 {
                          }
                        }
                      }
                      frame True {
                        n239 = call "加标仪器启动命令 (子VI).vi"("启动命令"=enum16{"启动水样流程", "启动加标流程", "排液", "停止"}."排液", "仪器"=enum16{"", "氨氮", "总磷", "总氮", "CODMn", "CODCr"}."总氮") -> ()  [unwired: 9 in, 1 out]
                        n240 = global read "与总氮交互全局.vi" "总氮测量数据区"() -> (w252:T12)
                        n241 = Unbundle By Name(w252) -> ("水样数据时间"=w255:timestamp, "水样实测值"=w256:sgl)
                        n242 = global read "平行样测试全局变量.vi" "总氮"() -> (w253:T10)
                        n243 = Bundle By Name(cluster=w253, "第二次水样测试时间"=w255, "第二次水样浓度值"=w256) -> (w254:T10)
                        n244 = global write "平行样测试全局变量.vi" "总氮"(w254) -> ()
                      }
                    }
                  }
                  frame "存储平行样测试数据" {
                    n245 = global read "平行样测试全局变量.vi" "总氮"() -> (w258:T10)
                    n246 = call "平行样测试数据写入.vi"("data"=w258) -> ()  [unwired: 10 in, 1 out]
                  }
                  frame "结束" {
                  }
                }
                n247 = feedback-in #9(w153) -> ()
              }
            }
            n248 = case shown="真" w146 {
              tunnel: [TRUE w479] -> w144
              tunnel: w135 -> [_ w477]
              tunnel: w134 -> [_ w476]
              frame False {
              }
              frame True {
                # "总磷平行样流程"
                n249 = feedback #12(平行样测试流程."待机") -> (w481:T3)
                n250 = case shown="\"待机\", 默认" w481 {
                  tunnel: [w482 w492 w521 w535 w569 平行样测试流程."结束" 平行样测试流程."结束"] -> w480
                  tunnel: [_ _ _ _ _ _ TRUE] -> w479
                  tunnel: w477 -> [_ w504 _ w537 _ _ _]
                  tunnel: w476 -> [_ w503 _ w536 _ _ _]
                  frame "待机", Default {
                    n251 = global read "加标回收状态全局变量.vi" "总磷状态"() -> (w486:u16)
                    n252 = case shown="0" w486 {
                      tunnel: [FALSE ("s") FALSE ("s") TRUE ("s")] -> w485
                      frame 0 {
                        n253 = call "加标仪器启动命令 (子VI).vi"("启动命令"=enum16{"启动水样流程", "启动加标流程", "排液", "停止"}."启动水样流程", "仪器"=enum16{"", "氨氮", "总磷", "总氮", "CODMn", "CODCr"}."总磷") -> ()  [unwired: 9 in, 1 out]
                      }
                      frame 1, Default {
                      }
                      frame 5 {
                      }
                    }
                    n254 = Select(t=平行样测试流程."第一次水样测试启动", s=w485, f=平行样测试流程."待机") -> (s? t:f=w482:T3)
                  }
                  frame "第一次水样测试启动" {
                    n255 = call "总磷启动命令.vi"("参数"=T4 {"站号"=1, "量程切换"=enum."AUTO", "控制命令"=enum."启动测量", "模式设置"=enum."受控模式", "测量间隔"=0}) -> ("启动命令"=w502:cluster{"命令":string, "data":variant})  [unwired: 10 in]
                    n256 = Enqueue Element(queue=w504, element=w502, error in (no error)=w503) -> (error out=w493:errorcluster)  [unwired: 1 in, 2 out]
                    n257 = feedback #13() -> (w497:i32)  [unwired: 1 in]
                    n258 = Increment(x=w497) -> (x+1=w496:i32)
                    n259 = First Call?() -> (First Call?: T/F=w498:bool)
                    n260 = Select(t=0, s=w498, f=w496) -> (s? t:f=w495:i32)
                    n261 = feedback-in #13(w495) -> ()
                    n262 = Greater Or Equal?(x=w495, y=60) -> (x >= y?=w500:bool)
                    n263 = case shown="假" w500 {
                      tunnel: [w509 平行样测试流程."结束"] -> w492
                      tunnel: w493 -> [_ _]
                      frame False {
                        n264 = global read "与总磷交互全局.vi" "总磷状态告警区"() -> (w505:T11)
                        n265 = Unbundle By Name(w505) -> ("工作状态"=w506:T6)
                        n266 = Not Equal To 0?(x=w506) -> (x != 0?=w510:bool)
                        n267 = Select(t=平行样测试流程."第一次水样测试中", s=w510, f=平行样测试流程."第一次水样测试启动") -> (s? t:f=w509:T3)
                      }
                      frame True {
                        n268 = Get Date/Time In Seconds() -> (seconds since 1Jan1904=w513:timestamp)
                        n269 = Bundle By Name(cluster=T5 {"时间标识"=timestamp(0 s since 1904-01-01), "设备"="", "日志信息"=""} ("data in"), "时间标识"=w513, "设备"="总磷", "日志信息"="总磷水样启动失败") -> (w511:T5)
                        n270 = call "质控报警信息.vi"("data in"=w511) -> ()  [unwired: 10 in, 1 out]
                      }
                    }
                  }
                  frame "第一次水样测试中" {
                    n271 = global read "与总磷交互全局.vi" "总磷状态告警区"() -> (w517:T11)
                    n272 = Unbundle By Name(w517) -> ("工作状态"=w520:T6)
                    n273 = Equal?(x=w520, y=T6."空闲" ("工作状态")) -> (x = y?=w518:bool)
                    n274 = case shown="真" w518 {
                      tunnel: [w522 平行样测试流程."第二次水样测试启动"] -> w521
                      frame False {
                        n275 = flat-sequence {
                          tunnel: [平行样测试流程."第一次水样测试中"] -> w522
                          frame #0 {
                            n276 = Wait (ms)(milliseconds to wait=u32 1000 ("等待时间（毫秒）")) -> ()  [unwired: 1 out]
                          }
                          frame #1 {
                          }
                        }
                      }
                      frame True {
                        n277 = call "加标仪器启动命令 (子VI).vi"("启动命令"=enum16{"启动水样流程", "启动加标流程", "排液", "停止"}."排液", "仪器"=enum16{"", "氨氮", "总磷", "总氮", "CODMn", "CODCr"}."总磷") -> ()  [unwired: 9 in, 1 out]
                        n278 = global read "与总磷交互全局.vi" "总磷测量数据区"() -> (w527:T12)
                        n279 = Unbundle By Name(w527) -> ("水样数据时间"=w530:timestamp, "水样实测值"=w531:sgl)
                        n280 = global read "平行样测试全局变量.vi" "总磷"() -> (w528:T10)
                        n281 = Bundle By Name(cluster=w528, "时间标识"=w530, "第一次水样浓度值"=w531) -> (w529:T10)
                        n282 = global write "平行样测试全局变量.vi" "总磷"(w529) -> ()
                      }
                    }
                  }
                  frame "第二次水样测试启动" {
                    n283 = global read "加标回收状态全局变量.vi" "总磷状态"() -> (w534:u16)
                    n284 = case shown="0" w534 {
                      tunnel: [FALSE ("s") FALSE ("s") TRUE ("s")] -> w533
                      frame 0 {
                        n285 = call "加标仪器启动命令 (子VI).vi"("启动命令"=enum16{"启动水样流程", "启动加标流程", "排液", "停止"}."启动水样流程", "仪器"=enum16{"", "氨氮", "总磷", "总氮", "CODMn", "CODCr"}."总磷") -> ()  [unwired: 9 in, 1 out]
                      }
                      frame 1, Default {
                      }
                      frame 5 {
                      }
                    }
                    n286 = case shown="假" w533 {
                      tunnel: w537 -> [_ w546]
                      tunnel: w536 -> [_ w545]
                      tunnel: [平行样测试流程."第二次水样测试启动" w544] -> w535
                      frame False {
                      }
                      frame True {
                        n287 = call "总磷启动命令.vi"("参数"=T4 {"站号"=1, "量程切换"=enum."AUTO", "控制命令"=enum."启动测量", "模式设置"=enum."受控模式", "测量间隔"=0}) -> ("启动命令"=w556:cluster{"命令":string, "data":variant})  [unwired: 10 in]
                        n288 = Enqueue Element(queue=w546, element=w556, error in (no error)=w545) -> (error out=w547:errorcluster)  [unwired: 1 in, 2 out]
                        n289 = feedback #14() -> (w551:i32)  [unwired: 1 in]
                        n290 = Increment(x=w551) -> (x+1=w550:i32)
                        n291 = First Call?() -> (First Call?: T/F=w552:bool)
                        n292 = Select(t=0, s=w552, f=w550) -> (s? t:f=w549:i32)
                        n293 = feedback-in #14(w549) -> ()
                        n294 = Greater Or Equal?(x=w549, y=60) -> (x >= y?=w554:bool)
                        n295 = case shown="假" w554 {
                          tunnel: [w561 平行样测试流程."结束"] -> w544
                          tunnel: w547 -> [_ _]
                          frame False {
                            n296 = global read "与总磷交互全局.vi" "总磷状态告警区"() -> (w557:T11)
                            n297 = Unbundle By Name(w557) -> ("工作状态"=w558:T6)
                            n298 = Not Equal To 0?(x=w558) -> (x != 0?=w562:bool)
                            n299 = Select(t=平行样测试流程."第二次水样测试中", s=w562, f=平行样测试流程."第二次水样测试启动") -> (s? t:f=w561:T3)
                          }
                          frame True {
                            n300 = Get Date/Time In Seconds() -> (seconds since 1Jan1904=w565:timestamp)
                            n301 = Bundle By Name(cluster=T5 {"时间标识"=timestamp(0 s since 1904-01-01), "设备"="", "日志信息"=""} ("data in"), "时间标识"=w565, "设备"="总磷", "日志信息"="总磷水样启动失败") -> (w563:T5)
                            n302 = call "质控报警信息.vi"("data in"=w563) -> ()  [unwired: 10 in, 1 out]
                          }
                        }
                      }
                    }
                  }
                  frame "第二次水样测试中" {
                    n303 = global read "与总磷交互全局.vi" "总磷状态告警区"() -> (w570:T11)
                    n304 = Unbundle By Name(w570) -> ("工作状态"=w573:T6)
                    n305 = Equal?(x=w573, y=T6."空闲" ("工作状态")) -> (x = y?=w571:bool)
                    n306 = case shown="真" w571 {
                      tunnel: [w574 平行样测试流程."存储平行样测试数据"] -> w569
                      frame False {
                        n307 = flat-sequence {
                          tunnel: [平行样测试流程."第二次水样测试中"] -> w574
                          frame #0 {
                            n308 = Wait (ms)(milliseconds to wait=u32 1000 ("等待时间（毫秒）")) -> ()  [unwired: 1 out]
                          }
                          frame #1 {
                          }
                        }
                      }
                      frame True {
                        n309 = call "加标仪器启动命令 (子VI).vi"("启动命令"=enum16{"启动水样流程", "启动加标流程", "排液", "停止"}."排液", "仪器"=enum16{"", "氨氮", "总磷", "总氮", "CODMn", "CODCr"}."总磷") -> ()  [unwired: 9 in, 1 out]
                        n310 = global read "与总磷交互全局.vi" "总磷测量数据区"() -> (w579:T12)
                        n311 = Unbundle By Name(w579) -> ("水样数据时间"=w582:timestamp, "水样实测值"=w583:sgl)
                        n312 = global read "平行样测试全局变量.vi" "总磷"() -> (w580:T10)
                        n313 = Bundle By Name(cluster=w580, "第二次水样测试时间"=w582, "第二次水样浓度值"=w583) -> (w581:T10)
                        n314 = global write "平行样测试全局变量.vi" "总磷"(w581) -> ()
                      }
                    }
                  }
                  frame "存储平行样测试数据" {
                    n315 = global read "平行样测试全局变量.vi" "总磷"() -> (w585:T10)
                    n316 = call "平行样测试数据写入.vi"("data"=w585) -> ()  [unwired: 10 in, 1 out]
                  }
                  frame "结束" {
                  }
                }
                n317 = feedback-in #12(w480) -> ()
              }
            }
            n318 = case shown="真" w142 {
              tunnel: [TRUE w360] -> w141
              frame False {
              }
              frame True {
                # "CODCr平行样流程"
                n319 = feedback #15(平行样测试流程."待机") -> (w362:T3)
                n320 = case shown="\"待机\", 默认" w362 {
                  tunnel: [w363 w383 w405 w419 w458 平行样测试流程."结束" 平行样测试流程."结束"] -> w361
                  tunnel: [_ _ _ _ _ _ TRUE] -> w360
                  frame "待机", Default {
                    n321 = global read "加标回收状态全局变量.vi" "CODCr状态"() -> (w367:u16)
                    n322 = case shown="0" w367 {
                      tunnel: [FALSE ("s") FALSE ("s") TRUE ("s")] -> w366
                      frame 0 {
                        n323 = call "加标仪器启动命令 (子VI).vi"("启动命令"=enum16{"启动水样流程", "启动加标流程", "排液", "停止"}."启动水样流程", "仪器"=enum16{"", "氨氮", "总磷", "总氮", "CODMn", "CODCr"}."CODCr") -> ()  [unwired: 9 in, 1 out]
                      }
                      frame 1, Default {
                      }
                      frame 5 {
                      }
                    }
                    n324 = Select(t=平行样测试流程."第一次水样测试启动", s=w366, f=平行样测试流程."待机") -> (s? t:f=w363:T3)
                  }
                  frame "第一次水样测试启动" {
                    n325 = call "CODCr启动命令 (子VI).vi"("启动测量模式"=T7 {"测量模式"=enum."水样测量"}) -> ("错误输出"=w373:errorcluster)  [unwired: 10 in]
                    n326 = First Call?() -> (First Call?: T/F=w375:bool)
                    n327 = case shown="真" w375 {
                      frame False {
                      }
                      frame True {
                        n328 = Get Date/Time In Seconds() -> (seconds since 1Jan1904=w386:timestamp)
                        n329 = Bundle By Name(cluster=T8 {"时间标识"=timestamp(0 s since 1904-01-01), "设备"="", "日志信息"="", "流程参数"=""} ("data in"), "时间标识"=w386, "设备"="CODCr", "日志信息"="-->>CODCr启动水样") -> (w387:T8)
                        n330 = call "质控日志存储 (子VI).vi"("data in"=w387) -> ()  [unwired: 11 in]
                      }
                    }
                    n331 = feedback #16() -> (w379:i32)  [unwired: 1 in]
                    n332 = Increment(x=w379) -> (x+1=w380:i32)
                    n333 = First Call?() -> (First Call?: T/F=w378:bool)
                    n334 = Select(t=0, s=w378, f=w380) -> (s? t:f=w381:i32)
                    n335 = feedback-in #16(w381) -> ()
                    n336 = Greater Or Equal?(x=w381, y=60) -> (x >= y?=w376:bool)
                    n337 = case shown="真" w376 {
                      tunnel: [w393 平行样测试流程."结束"] -> w383
                      tunnel: w373 -> [_ _]
                      frame False {
                        n338 = global read "与CODCr交互全局.vi" "CODCr状态告警区"() -> (w390:T11)
                        n339 = Unbundle By Name(w390) -> ("工作状态"=w389:T6)
                        n340 = Not Equal To 0?(x=w389) -> (x != 0?=w394:bool)
                        n341 = Select(t=平行样测试流程."第一次水样测试中", s=w394, f=平行样测试流程."第一次水样测试启动") -> (s? t:f=w393:T3)
                      }
                      frame True {
                        n342 = Get Date/Time In Seconds() -> (seconds since 1Jan1904=w397:timestamp)
                        n343 = Bundle By Name(cluster=T5 {"时间标识"=timestamp(0 s since 1904-01-01), "设备"="", "日志信息"=""} ("data in"), "时间标识"=w397, "设备"="CODCr", "日志信息"="CODCr水样启动失败") -> (w395:T5)
                        n344 = call "质控报警信息.vi"("data in"=w395) -> ()  [unwired: 10 in, 1 out]
                      }
                    }
                  }
                  frame "第一次水样测试中" {
                    n345 = global read "与CODCr交互全局.vi" "CODCr状态告警区"() -> (w404:T11)
                    n346 = Unbundle By Name(w404) -> ("工作状态"=w401:T6)
                    n347 = Equal?(x=w401, y=T6."空闲" ("工作状态")) -> (x = y?=w403:bool)
                    n348 = case shown="真" w403 {
                      tunnel: [w406 平行样测试流程."第二次水样测试启动"] -> w405
                      frame False {
                        n349 = flat-sequence {
                          tunnel: [平行样测试流程."第一次水样测试中"] -> w406
                          frame #0 {
                            n350 = Wait (ms)(milliseconds to wait=u32 1000 ("等待时间（毫秒）")) -> ()  [unwired: 1 out]
                          }
                          frame #1 {
                          }
                        }
                      }
                      frame True {
                        n351 = global read "与CODCr交互全局.vi" "CODCr测量数据区"() -> (w413:T12)
                        n352 = Unbundle By Name(w413) -> ("水样数据时间"=w412:timestamp, "水样实测值"=w411:sgl)
                        n353 = global read "平行样测试全局变量.vi" "CODcr"() -> (w415:T10)
                        n354 = Bundle By Name(cluster=w415, "时间标识"=w412, "第一次水样浓度值"=w411) -> (w414:T10)
                        n355 = global write "平行样测试全局变量.vi" "CODcr"(w414) -> ()
                        n356 = call "加标仪器启动命令 (子VI).vi"("启动命令"=enum16{"启动水样流程", "启动加标流程", "排液", "停止"}."排液", "仪器"=enum16{"", "氨氮", "总磷", "总氮", "CODMn", "CODCr"}."CODCr") -> ()  [unwired: 9 in, 1 out]
                      }
                    }
                  }
                  frame "第二次水样测试启动" {
                    n357 = global read "加标回收状态全局变量.vi" "CODCr状态"() -> (w418:u16)
                    n358 = case shown="0" w418 {
                      tunnel: [FALSE ("s") FALSE ("s") TRUE ("s")] -> w417
                      frame 0 {
                        n359 = call "加标仪器启动命令 (子VI).vi"("启动命令"=enum16{"启动水样流程", "启动加标流程", "排液", "停止"}."启动水样流程", "仪器"=enum16{"", "氨氮", "总磷", "总氮", "CODMn", "CODCr"}."CODCr") -> ()  [unwired: 9 in, 1 out]
                      }
                      frame 1, Default {
                      }
                      frame 5 {
                      }
                    }
                    n360 = case shown="假" w417 {
                      tunnel: [平行样测试流程."第二次水样测试启动" w436] -> w419
                      frame False {
                      }
                      frame True {
                        n361 = First Call?() -> (First Call?: T/F=w431:bool)
                        n362 = feedback #17() -> (w432:i32)  [unwired: 1 in]
                        n363 = Increment(x=w432) -> (x+1=w433:i32)
                        n364 = Select(t=0, s=w431, f=w433) -> (s? t:f=w434:i32)
                        n365 = feedback-in #17(w434) -> ()
                        n366 = call "CODCr启动命令 (子VI).vi"("启动测量模式"=T7 {"测量模式"=enum."水样测量"}) -> ("错误输出"=w426:errorcluster)  [unwired: 10 in]
                        n367 = Greater Or Equal?(x=w434, y=60) -> (x >= y?=w429:bool)
                        n368 = First Call?() -> (First Call?: T/F=w428:bool)
                        n369 = case shown="假" w429 {
                          tunnel: [w446 平行样测试流程."结束"] -> w436
                          tunnel: w426 -> [_ _]
                          frame False {
                            n370 = global read "与CODCr交互全局.vi" "CODCr状态告警区"() -> (w443:T11)
                            n371 = Unbundle By Name(w443) -> ("工作状态"=w442:T6)
                            n372 = Not Equal To 0?(x=w442) -> (x != 0?=w447:bool)
                            n373 = Select(t=平行样测试流程."第二次水样测试中", s=w447, f=平行样测试流程."第二次水样测试启动") -> (s? t:f=w446:T3)
                          }
                          frame True {
                            n374 = Get Date/Time In Seconds() -> (seconds since 1Jan1904=w450:timestamp)
                            n375 = Bundle By Name(cluster=T5 {"时间标识"=timestamp(0 s since 1904-01-01), "设备"="", "日志信息"=""} ("data in"), "时间标识"=w450, "设备"="CODCr", "日志信息"="CODCr启动失败") -> (w448:T5)
                            n376 = call "质控报警信息.vi"("data in"=w448) -> ()  [unwired: 10 in, 1 out]
                          }
                        }
                        n377 = case shown="真" w428 {
                          frame False {
                          }
                          frame True {
                            n378 = Get Date/Time In Seconds() -> (seconds since 1Jan1904=w439:timestamp)
                            n379 = Bundle By Name(cluster=T8 {"时间标识"=timestamp(0 s since 1904-01-01), "设备"="", "日志信息"="", "流程参数"=""} ("data in"), "时间标识"=w439, "设备"="CODCr", "日志信息"="-->>CODCr启动水样") -> (w440:T8)
                            n380 = call "质控日志存储 (子VI).vi"("data in"=w440) -> ()  [unwired: 11 in]
                          }
                        }
                      }
                    }
                  }
                  frame "第二次水样测试中" {
                    n381 = global read "与CODCr交互全局.vi" "CODCr状态告警区"() -> (w457:T11)
                    n382 = Unbundle By Name(w457) -> ("工作状态"=w454:T6)
                    n383 = Equal?(x=w454, y=T6."空闲" ("工作状态")) -> (x = y?=w456:bool)
                    n384 = case shown="真" w456 {
                      tunnel: [w459 平行样测试流程."存储平行样测试数据"] -> w458
                      frame False {
                        n385 = flat-sequence {
                          tunnel: [平行样测试流程."第二次水样测试中"] -> w459
                          frame #0 {
                            n386 = Wait (ms)(milliseconds to wait=u32 1000 ("等待时间（毫秒）")) -> ()  [unwired: 1 out]
                          }
                          frame #1 {
                          }
                        }
                      }
                      frame True {
                        n387 = global read "与CODCr交互全局.vi" "CODCr测量数据区"() -> (w466:T12)
                        n388 = Unbundle By Name(w466) -> ("水样数据时间"=w465:timestamp, "水样实测值"=w464:sgl)
                        n389 = global read "平行样测试全局变量.vi" "CODcr"() -> (w468:T10)
                        n390 = Bundle By Name(cluster=w468, "第二次水样测试时间"=w465, "第二次水样浓度值"=w464) -> (w467:T10)
                        n391 = global write "平行样测试全局变量.vi" "CODcr"(w467) -> ()
                        n392 = call "加标仪器启动命令 (子VI).vi"("启动命令"=enum16{"启动水样流程", "启动加标流程", "排液", "停止"}."排液", "仪器"=enum16{"", "氨氮", "总磷", "总氮", "CODMn", "CODCr"}."CODCr") -> ()  [unwired: 9 in, 1 out]
                      }
                    }
                  }
                  frame "存储平行样测试数据" {
                    n393 = global read "平行样测试全局变量.vi" "CODcr"() -> (w470:T10)
                    n394 = call "平行样测试数据写入.vi"("data"=w470) -> ()  [unwired: 10 in, 1 out]
                  }
                  frame "结束" {
                    n395 = First Call?() -> (First Call?: T/F=w473:bool)
                    n396 = case shown="真" w473 {
                      frame False {
                      }
                      frame True {
                        (unwired) "-->>CODCr停止" ("日志信息")
                        (unwired) "CODCr" ("设备")
                        n397 = call "质控日志存储 (子VI).vi"() -> ()  [unwired: 12 in]
                      }
                    }
                  }
                }
                n398 = feedback-in #15(w361) -> ()
              }
            }
            n399 = Compound Arithmetic op=AND ("复合运算")(w145, w141, w144, w140, w138) -> (w131:bool)
          }
        }
        n400 = case shown="假" w96 {
          tunnel: w114 -> [w117 w126]
          tunnel: [w116 w125] -> w112
          tunnel: w94 -> [w115 _]
          frame False {
            n401 = Select(t=enum16{"初始化", "采配水启动", "等待", "配水", "排水", "结束"}."结束" ("枚举"), s=w115, f=w117) -> (s? t:f=w116:enum16{"初始化", "采配水启动", "等待", "配水", "排水", "结束"})
          }
          frame True {
            n402 = global read "与采配水交互全局.vi" "状态"() -> (w124:T9)
            n403 = Unbundle By Name(w124) -> ("R0"=w123:i16)
            n404 = Equal To 0?(x=w123) -> (x = 0?=w120:bool)
            n405 = Greater?(x=w123, y=i16 6) -> (0:w121:bool)
            n406 = Or(x=w120, y=w121) -> (x .or. y?=w119:bool)
            n407 = Select(t=enum16{"初始化", "采配水启动", "等待", "配水", "排水", "结束"}."排水" ("枚举"), s=w119, f=w126) -> (s? t:f=w125:enum16{"初始化", "采配水启动", "等待", "配水", "排水", "结束"})
          }
        }
        n408 = Select(t=enum16{"初始化", "采配水启动", "等待", "配水", "排水", "结束"}."结束", s=w95, f=w112) -> (s? t:f=w111:enum16{"初始化", "采配水启动", "等待", "配水", "排水", "结束"})
      }
      frame "排水" {
        n409 = Increment(x=w707) -> (x+1=w703:enum16{"初始化", "采配水启动", "等待", "配水", "排水", "结束"})
        n410 = Enqueue Element At Opposite End(queue=w708, element=T2 {"命令"="单个写入", {"starting address"=303, "holding register value"=1}} ("元素")) -> ()  [unwired: 2 in, 3 out]
        n411 = Select(t=enum16{"初始化", "采配水启动", "等待", "配水", "排水", "结束"}."结束", s=w704, f=w703) -> (s? t:f=w702:enum16{"初始化", "采配水启动", "等待", "配水", "排水", "结束"})
      }
      frame "结束" {
        n412 = Increment(x=w714) -> (x+1=w713:enum16{"初始化", "采配水启动", "等待", "配水", "排水", "结束"})
        n413 = global write "质控测完标志全局 1.vi" "质控流程中"(FALSE ("质控流程中")) -> ()
      }
    }
    "枚举" <- w39
    n414 = Format Into String(format string="%s,当前运行时间%d秒" ("格式字符串"), w33, w32) -> ()  [unwired: 2 in, 2 out]
  }
  n415 = Cancel Notification(0:w15) -> (8:w14:refnum<notifier>)  [unwired: 1 in, 2 out]
  n416 = Release Notifier(notifier=w14) -> ()  [unwired: 2 in, 3 out]
